vi "task 1.vi"() -> ()   [LabVIEW 2017]
panel:
  out "h value":dbl
  in  "h setting":dbl(knob) scale=0.0..10.0
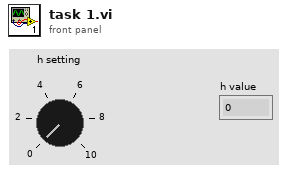
[diagram p1: front panel]
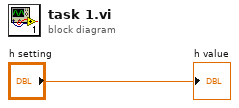
[diagram p0: block diagram]
diagram:
  "h value" <- "h setting"
